vi "PH_Cont-601k_PSU.check allowness for Flash Interval Setting.vi"(1 "Configuration":T1 items=["Ch intl, Fl intl, QSw intl", "Ch intl, Fl intl, QSw ext", "Ch intl, Fl ext, QSw intl", "Ch intl, Fl ext, QSw ext", "Ch ext, Fl int, QSw int", "Ch ext, Fl int, QSw ext", "Ch ext, Fl ext, QSw int", "Ch ext, Fl ext, QSw ext"]) -> (0 "Flash Interval Setting allowed?":bool)   [LabVIEW 2014, in "PH_Cont-601k_PSU.lvlib"]
uses:
  PH_Cont-601k_PSU.lvlib
  PH_Cont-601k_PSU.Configuration.ctl
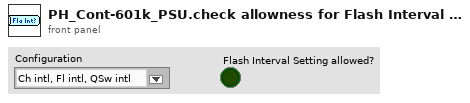
[diagram p1: front panel]
types:
  T1 = typedef "PH_Cont-601k_PSU.lvlib/PH_Cont-601k_PSU.Configuration.ctl" = u16
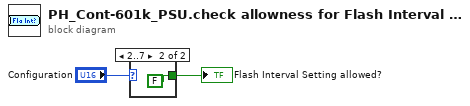
[diagram p0: block diagram]
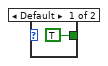
[diagram p2: hidden frame]
diagram:
  n1 = case shown="2..7" "Configuration" {
    tunnel: [TRUE FALSE] -> w2
    frame Default {
    }
    frame 2..7 {
    }
  }
  "Flash Interval Setting allowed?" <- w2
